vi "SECADO_JKI_v120.vi"() -> ()   [LabVIEW 2017] (continued)
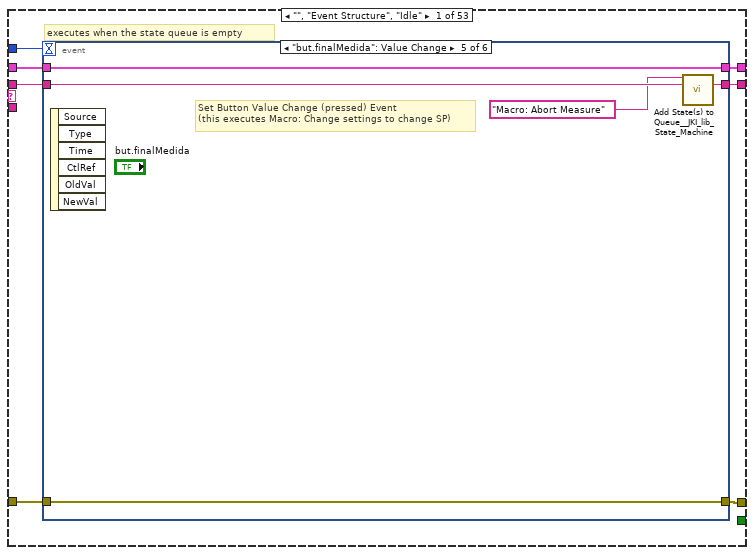
[diagram p2: hidden frame]
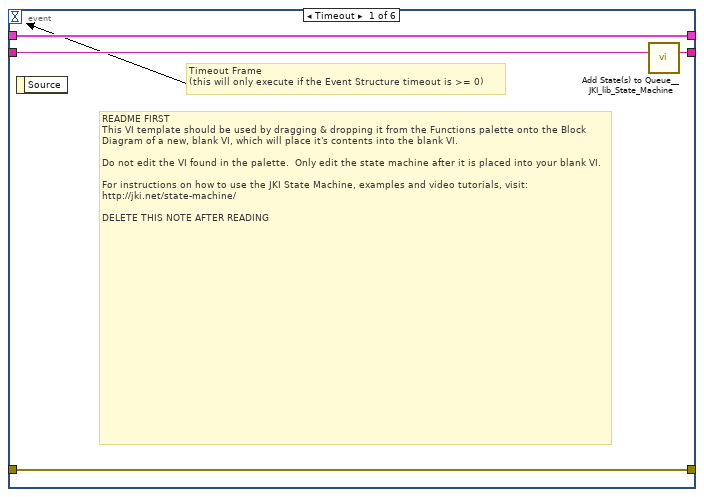
[diagram p3: hidden frame]
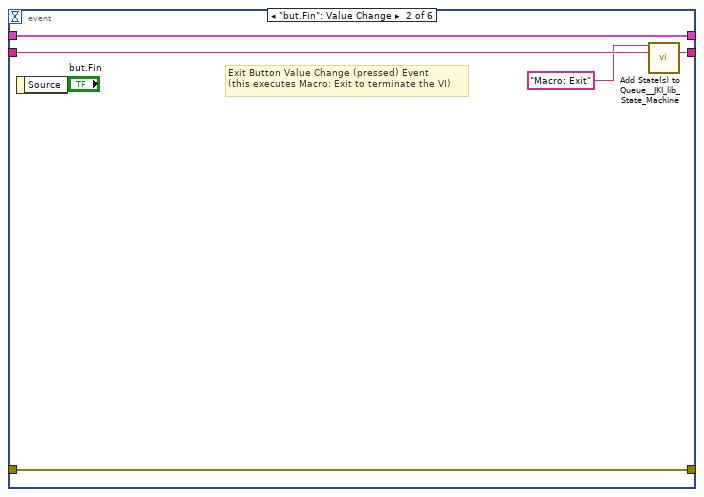
[diagram p4: hidden frame]
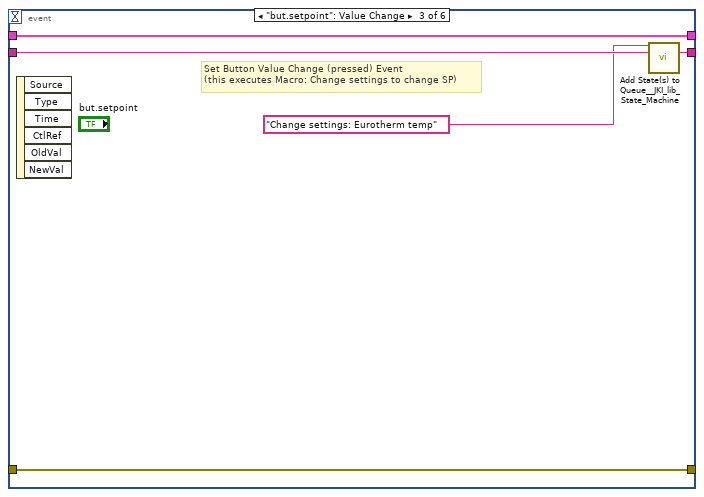
[diagram p5: hidden frame]
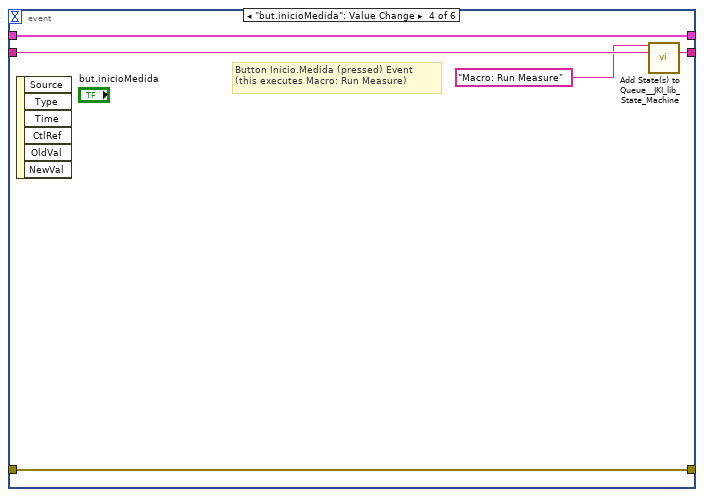
[diagram p6: hidden frame]
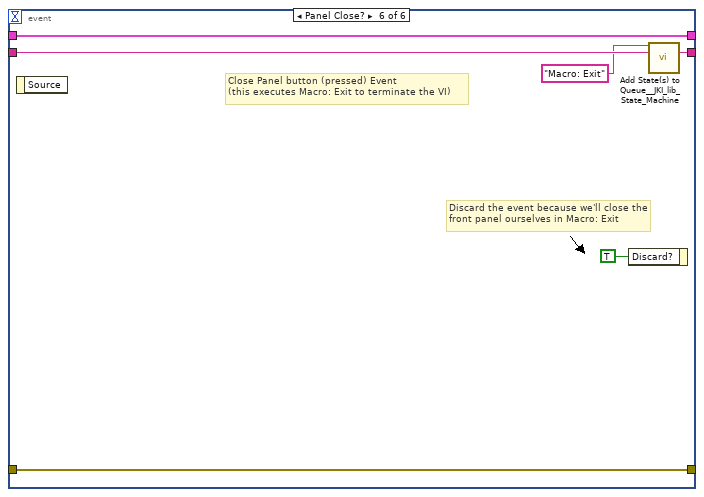
[diagram p7: hidden frame]
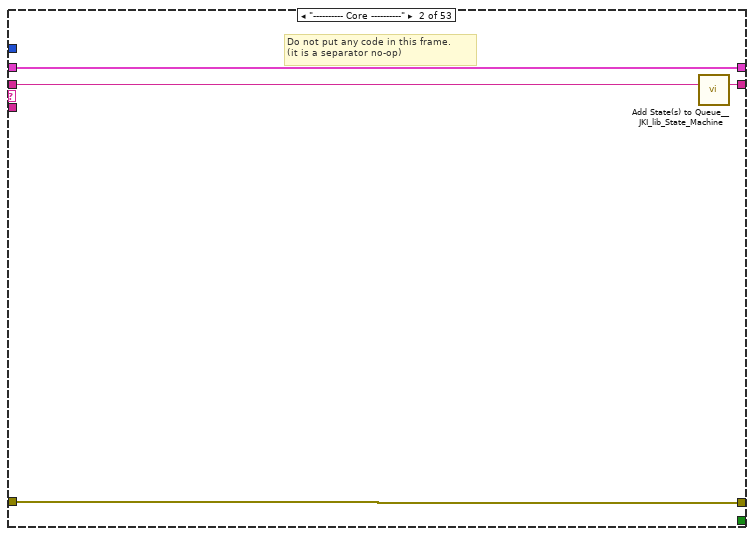
[diagram p8: hidden frame]
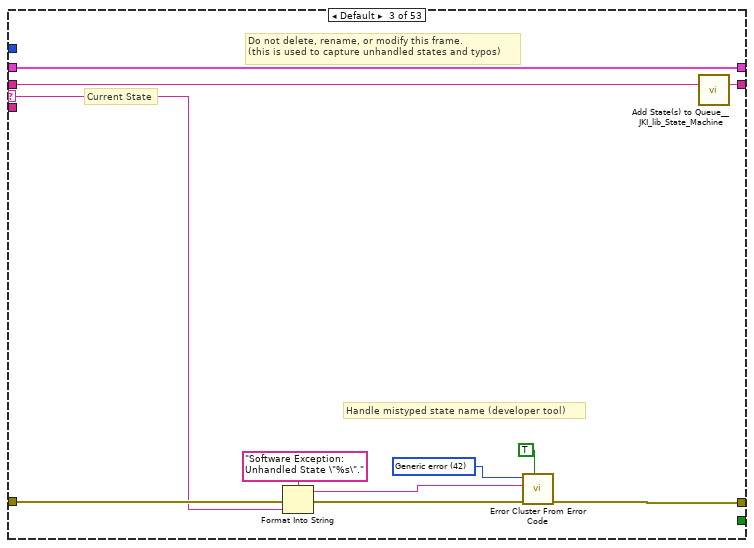
[diagram p9: hidden frame]
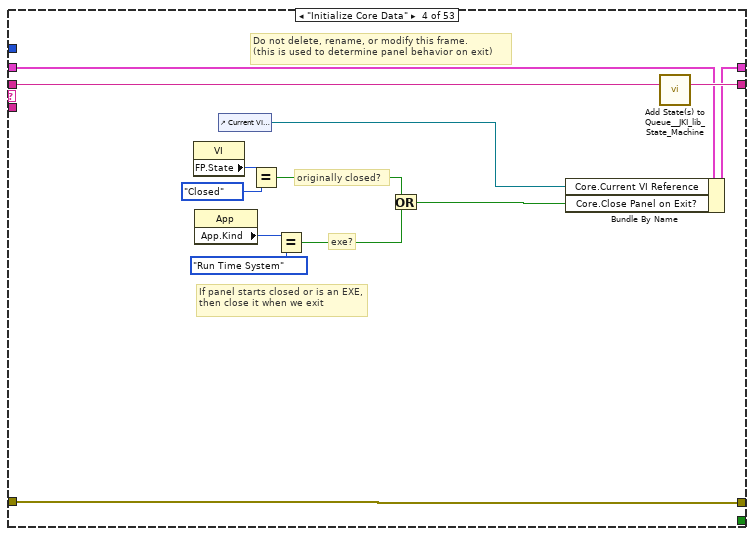
[diagram p10: hidden frame]
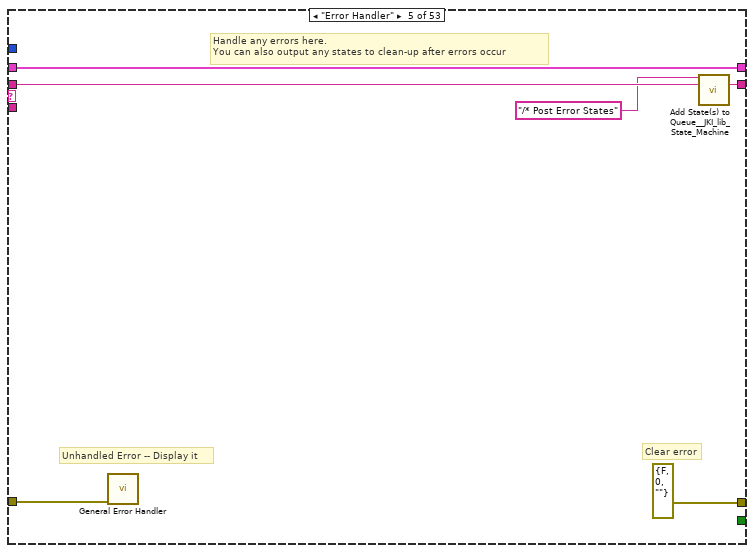
[diagram p11: hidden frame]
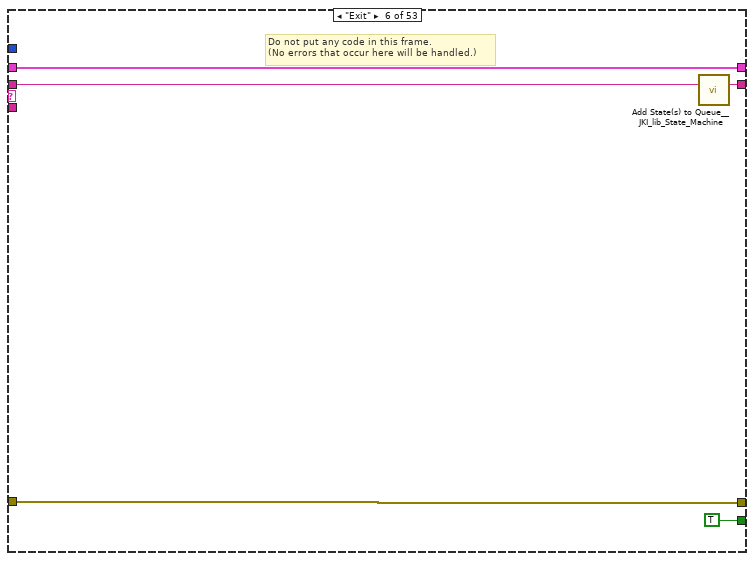
[diagram p12: hidden frame]
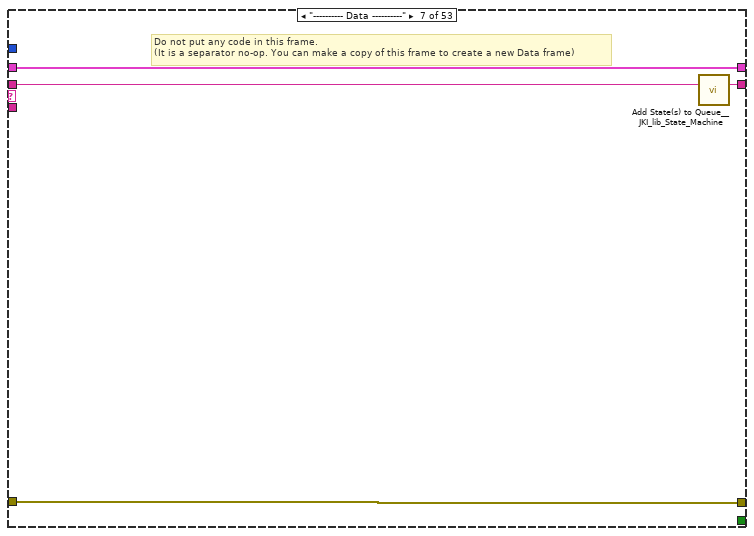
[diagram p13: hidden frame]
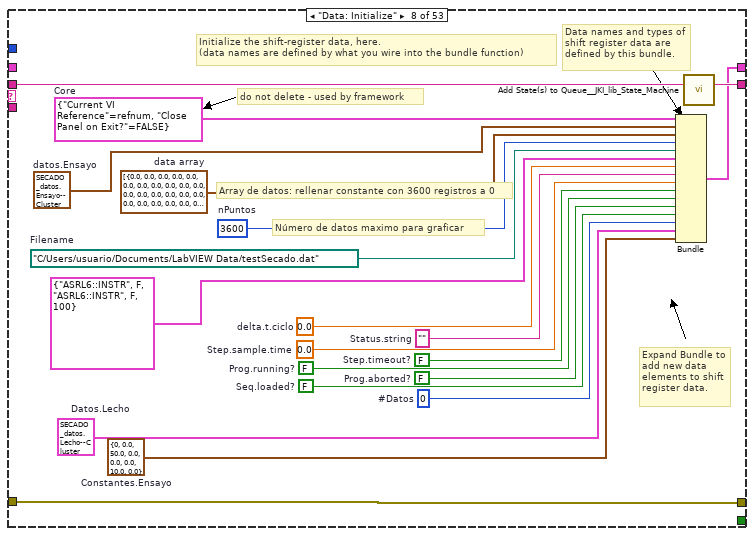
[diagram p14: hidden frame]
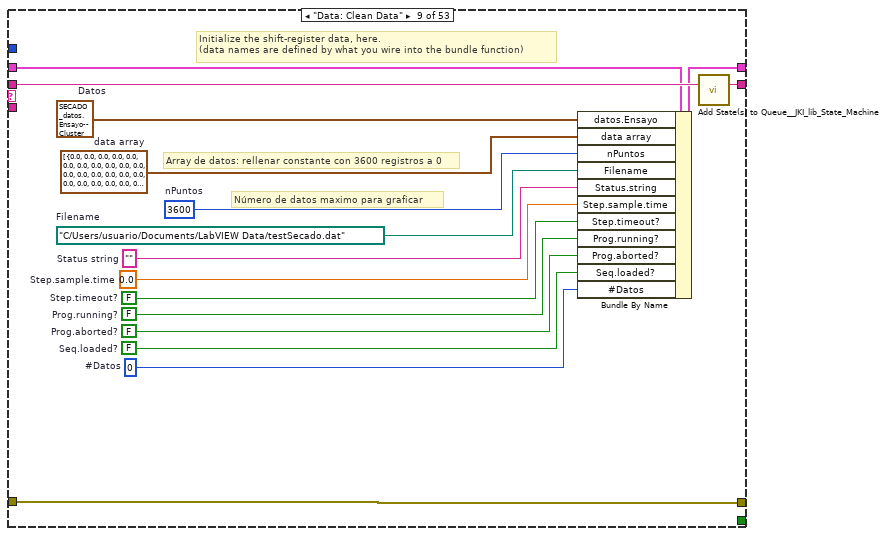
[diagram p15: hidden frame]
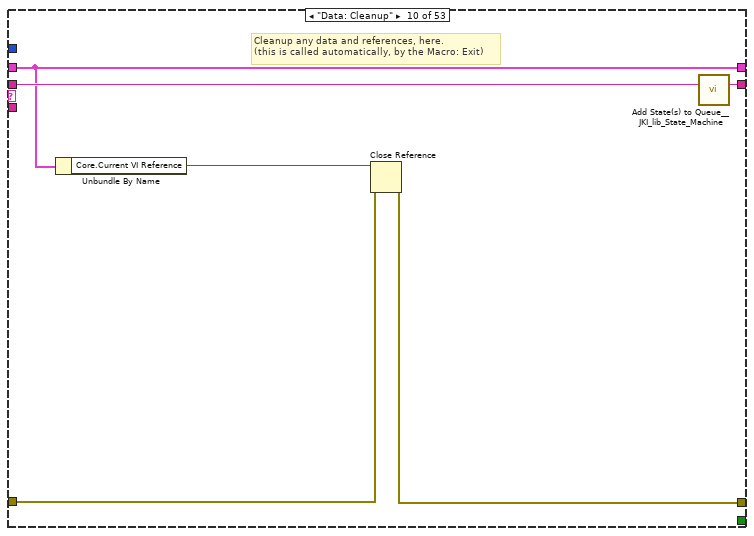
[diagram p16: hidden frame]
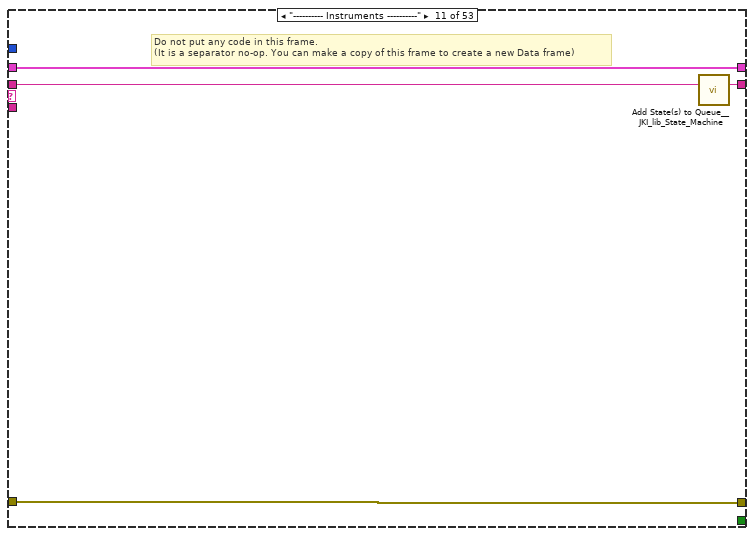
[diagram p17: hidden frame]
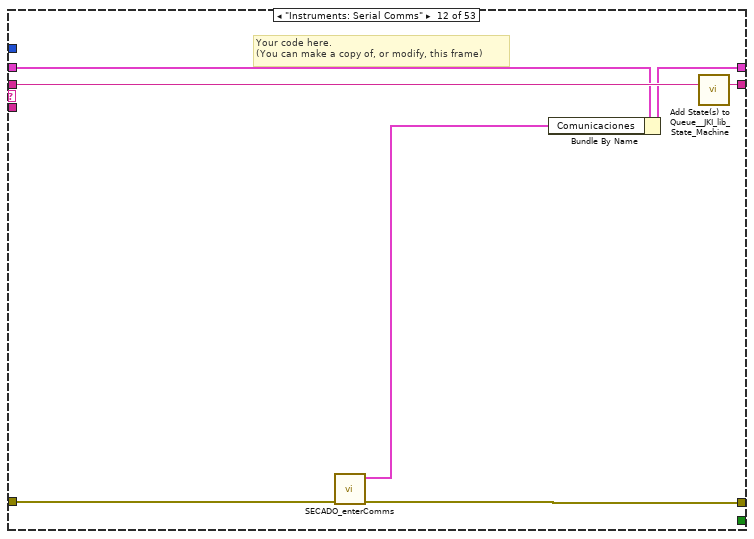
[diagram p18: hidden frame]
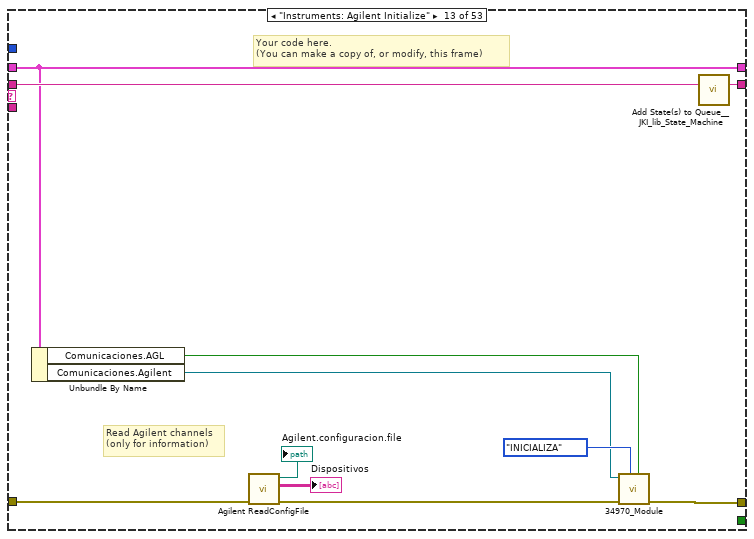
[diagram p19: hidden frame]
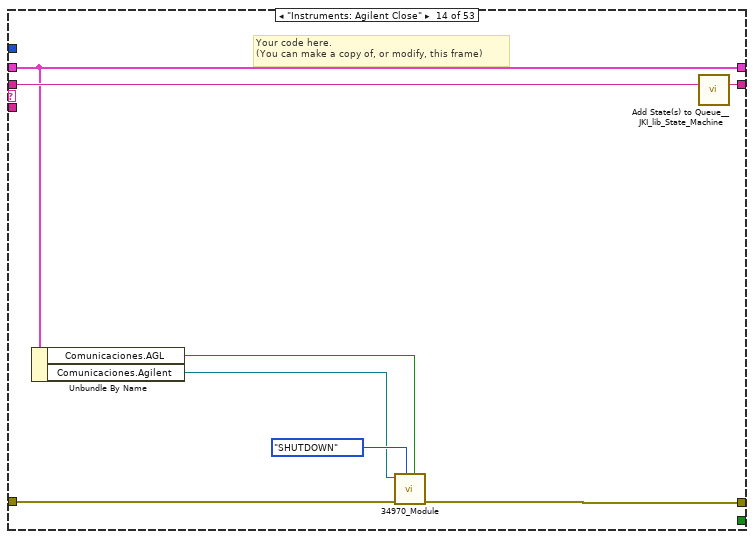
[diagram p20: hidden frame]
        n146 = Build Array(w405, w404, w403, w402) -> (→"EUROTHERM":cluster{dbl[], dbl[]}[])
        n147 = Build Array(w401, w400) -> (→"CAUDAL":cluster{dbl[], dbl[]}[])
        n148 = Build Array(w399) -> (→"POTENCIA CALEFACCION":cluster{dbl[], dbl[]}[])
        n149 = Build Array(w396, w395) -> (→"Q CEDIDO Y ABSORBIDO":cluster{dbl[], dbl[]}[])
        n150 = Build Array(w370, w369) -> (→"HUMEDAD":cluster{dbl[], dbl[]}[])
        n151 = Build Array(w368) -> (→"PRES_DIF":cluster{dbl[], dbl[]}[])
        n152 = Build Array(w388, w374, w373, w372, w371) -> (→"TEMPERATURA":cluster{dbl[], dbl[]}[])
        n153 = Build Array(w367, w360, w359) -> (→"VELOCIDAD AIRE":cluster{dbl[], dbl[]}[])
        n154 = Bundle By Name(cluster=w366, "data array"=w407) -> (w408:T19)
        n155 = call <vilib>:"Add State(s) to Queue__JKI_lib_State_Machine.vi"("State(s) in (\"\")"=w427) -> ("States Out"=w426:string)  [unwired: 14 in]
      }
      frame "---------- Macro ----------" {
        # "Do not put any code in this frame.\n(It is a separator no-op. You can make a copy of this frame to create a new Macro frame)"
        n156 = call <vilib>:"Add State(s) to Queue__JKI_lib_State_Machine.vi"("State(s) in (\"\")"=w455) -> ("States Out"=w454:string)  [unwired: 14 in]
      }
      frame "Macro: Inicializar" {
        w462 = "Data: Initialize\nData: Clean Data\nInitialize Core Data\nUI: Initialize\nUI: Front Panel State >> Open\nMacro: Interlock\nUI: Update Meas Data\nUI: Update Graphics\nInstruments: Serial Comms\nInstruments: Agilent Initialize\nInstruments: Eurotherm Initialize"  # Data: Initialize Data: Clean Data Initialize Core Data UI: Initialize UI: Front Panel State >> Open Macro: Interlock UI: Update Meas Data UI: Update Graphics Instruments: Serial Comms Instruments: Agilent Initialize Instruments: Eurotherm Initialize
        # "Initialization Macro\n(This is called once, when the VI starts)"
        n157 = Bundle By Name(cluster=w457, "Prog.running?"=TRUE ("Prog. Running?"), "Prog.aborted?"=FALSE ("Prog. Aborted?"), "Seq.loaded?"=FALSE ("Seq. Loaded?"), "Status.string"="Ready to start...") -> (w456:T19)
        n158 = call <vilib>:"Add State(s) to Queue__JKI_lib_State_Machine.vi"("State(s) in Front (\"\")"=w462, "State(s) in (\"\")"=w465) -> ("States Out"=w464:string)  [unwired: 13 in]
      }
      frame "Macro: Run Measure" {
        # "Run Measure Macro\n(This is called once, when the VI starts)"
        n159 = Bundle By Name(cluster=w472, "Prog.running?"=TRUE ("Prog. Running?"), "Prog.aborted?"=FALSE ("Prog. Aborted?"), "Seq.loaded?"=FALSE ("Seq. Loaded?"), "Status.string"="Adquisition in progress...") -> (w470:T19)
        n160 = call <vilib>:"Add State(s) to Queue__JKI_lib_State_Machine.vi"("State(s) in Front (\"\")"="UI: Initialize\nMacro: Interlock\nFile: Filename\nTiming: Initialize Total Time\nTiming: Initialize Sample Time\nMacro: Next Meas Cycle", "State(s) in (\"\")"=w475) -> ("States Out"=w474:string)  [unwired: 13 in]
      }
      frame "Macro: Abort Measure" {
        # "Abort Measure Macro\n(This is called when abort buton is pressed)"
        n161 = Bundle By Name(cluster=w480, "Prog.running?"=FALSE ("Prog. Running?"), "Prog.aborted?"=TRUE ("Prog. Aborted?"), "Seq.loaded?"=FALSE ("Seq. Loaded?"), "Status.string"="Adquisition aborted...") -> (w479:T19)
        n162 = One Button Dialog(message="Measure aborted") -> ()  [unwired: 1 in, 1 out]
        n163 = call <vilib>:"Add State(s) to Queue__JKI_lib_State_Machine.vi"("State(s) in (\"\")"="// Data: Set Seq. Aborted Flag >> True\n// Macro: Interlock\n// IO: Dwell  // finish current step (remove to abort immediately)\n// Data: Set Running Step >> -1\n// UI: Update Table Selection\n// Data: Set Seq. Aborted Flag >> False\nMacro: Interlock") -> ("States Out"=w485:string)  [unwired: 14 in]
      }
      frame "Macro: Next Meas Cycle" {
        # "Initialization Macro\n(This is called once, when the VI starts)"
        n164 = Unbundle By Name(w489) -> ("#Datos"=w487:i32)
        n165 = Increment(x=w487) -> (x+1=w486:i32)
        "#.datos" <- w486
        n166 = Bundle By Name(cluster=w489, "#Datos"=w486) -> (w488:T19)
        n167 = call <vilib>:"Add State(s) to Queue__JKI_lib_State_Machine.vi"("State(s) in Front (\"\")"="Timing: Measure Total Time\nMacro: Take Data\nMacro: Calculate\nMacro: Interlock\nFile: Save Data\nUI: Update Meas Data\nUI: Update Graphics\nSampling: Check For Next Sample", "State(s) in (\"\")"=w493) -> ("States Out"=w492:string)  [unwired: 13 in]
      }
      frame "Macro: Take Data" {
        # "Initialization Macro\n(This is called once, when the VI starts)"
        n168 = call <vilib>:"Add State(s) to Queue__JKI_lib_State_Machine.vi"("State(s) in Front (\"\")"="Measure data: Agilent Temp.PT100\nMeasure data: Agilent Temp.TERMOPAR\nMeasure data: Agilent Pressure\nMeasure data: Agilent Humidity\nMeasure data: Eurotherm Temperature", "State(s) in (\"\")"=w498) -> ("States Out"=w497:string)  [unwired: 13 in]
      }
      frame "Macro: Calculate" {
        # "Initialization Macro\n(This is called once, when the VI starts)"
        n169 = call <vilib>:"Add State(s) to Queue__JKI_lib_State_Machine.vi"("State(s) in Front (\"\")"="Calculations: Calculos 1", "State(s) in (\"\")"=w503) -> ("States Out"=w502:string)  [unwired: 13 in]
      }
      frame "Macro: Interlock" {
        # "Initialization Macro\n(This is called once, when the VI starts)"
        n170 = call <vilib>:"Add State(s) to Queue__JKI_lib_State_Machine.vi"("State(s) in Front (\"\")"="UI: Update Status\nUI: Update Interlock", "State(s) in (\"\")"=w508) -> ("States Out"=w507:string)  [unwired: 13 in]
      }
      frame "Macro: Exit" {
        # "Exit Macro\n(This is called once, when the VI exits)"
        n171 = Unbundle By Name(w516) -> ("Core.Close Panel on Exit?"=w515:bool)
        n172 = One Button Dialog(message="Program stop") -> ()  [unwired: 1 in, 1 out]
        n173 = Select(t="UI: Front Panel State >> Close", s=w515, f="") -> (s? t:f=w512:string)
        n174 = call <vilib>:"Add State(s) to Queue__JKI_lib_State_Machine.vi"("State(s) in (\"\")"=w512, "State(s) at Back (\"\")"="Data: Cleanup\nExit") -> ("States Out"=w510:string)  [unwired: 13 in]
        n175 = call <vilib>:"Add State(s) to Queue__JKI_lib_State_Machine.vi"("State(s) in Front (\"\")"=w510, "State(s) in (\"\")"=w519) -> ("States Out"=w518:string)  [unwired: 13 in]
      }
      frame "---------- File ----------" {
        # "Template Separator\n(You can make a copy of, or modify, this frame)"
        n176 = call <vilib>:"Add State(s) to Queue__JKI_lib_State_Machine.vi"("State(s) in (\"\")"=w523) -> ("States Out"=w522:string)  [unwired: 14 in]
      }
      frame "File: Filename" {
        # "Al arrancar la medida:\nHumedad.lecho = Humedad_inicial"
        # "Initialize and save head data"
        # "Your code here.\n(You can make a copy of, or modify, this frame)"
        n177 = call "SECADO_enterEnsayo.vi"("error in (no error)"=w530) -> ("error out"=w532:errorcluster, "Datos.Lecho"=w525:T5, "Constantes.Ensayo"=w526:T6)  [unwired: 7 in, 1 out]
        "Constantes.Ensayo" <- w526
        "Datos.Lecho" <- w525
        n178 = Unbundle By Name(w525) -> ("Hum_ini, f1"=w524:dbl)
        n179 = call "File_Module.vi"("Command"=File_Module_Control."Initialize", "error in (no error)"=w532, "Datos.Lecho"=w525, "Constantes.Ensayo"=w526) -> ("error out"=w529:errorcluster, "selected path"=w527:path)  [unwired: 6 in]
        "Fichero" <- w527
        n180 = Bundle By Name(cluster=w533, "Constantes.Ensayo"=w526, "Datos.Lecho"=w525, "Filename"=w527, "datos.Ensayo.Humedad.lecho, f1"=w524) -> (w528:T19)
        n181 = call <vilib>:"Add State(s) to Queue__JKI_lib_State_Machine.vi"("State(s) in (\"\")"=w535) -> ("States Out"=w534:string)  [unwired: 14 in]
      }
      frame "File: Save Data" {
        # "Your code here.\n(You can make a copy of, or modify, this frame)"
        n182 = Get Date/Time String() -> (date string=→"Fecha":string, time string=→"Hora":string)  [unwired: 3 in]
        n183 = Unbundle By Name(w538) -> ("datos.Ensayo"=w539:T4)
        n184 = call "File_Module.vi"("Command"=File_Module_Control."Save Data", "error in (no error)"=w541, "Datos.Ensayo"=w539) -> ("error out"=w540:errorcluster)  [unwired: 7 in, 1 out]
        n185 = call <vilib>:"Add State(s) to Queue__JKI_lib_State_Machine.vi"("State(s) in (\"\")"=w544) -> ("States Out"=w543:string)  [unwired: 14 in]
      }
      frame "---------- Sampling ----------" {
        # "Template Separator\n(You can make a copy of, or modify, this frame)"
        n186 = call <vilib>:"Add State(s) to Queue__JKI_lib_State_Machine.vi"("State(s) in (\"\")"=w548) -> ("States Out"=w547:string)  [unwired: 14 in]
      }
      frame "Sampling: Check For Next Sample" {
        # "Your code here.\n(You can make a copy of, or modify, this frame)"
        n187 = Unbundle By Name(w554) -> ("Step.timeout?"=w552:bool)
        n188 = Select(t="Timing: Initialize Sample Time\nMacro: Next Meas Cycle", s=w552, f="Idle  //Calls event structure\nTiming: Measure Sample Time\nSampling: Check For Next Sample // Come back here") -> (s? t:f=w550:string)
        n189 = call <vilib>:"Add State(s) to Queue__JKI_lib_State_Machine.vi"("State(s) in Front (\"\")"=w550, "State(s) in (\"\")"=w556) -> ("States Out"=w555:string)  [unwired: 13 in]
      }
      frame "---------- Measure data ----------" {
        # "Template Separator\n(You can make a copy of, or modify, this frame)"
        n190 = call <vilib>:"Add State(s) to Queue__JKI_lib_State_Machine.vi"("State(s) in (\"\")"=w560) -> ("States Out"=w559:string)  [unwired: 14 in]
      }
      frame "Measure data: Agilent Temp.PT100" {
        # "Agilent temperature readings code here.\n(You can make a copy of, or modify, this frame)"
        n191 = Unbundle By Name(w563) -> ("Comunicaciones.AGL"=w561:bool, "Comunicaciones.Agilent"=w562:refnum<visa-resource-name>)
        n192 = call "34970_Module.vi"("Agilent 34970A"=w561, "Command"=34970_Module_Control."LECTURA PT100", "error in (no error)"=w564, "VISA Agilent 34970A"=w562) -> ("error out"=w565:errorcluster, "TEMP.PT100"=w571:dbl[])  [unwired: 3 in, 3 out]
        n193 = Index Array(array=w571) -> (element #1=w569:dbl, element #2=w568:dbl, element #3=w567:dbl, element #4=w566:dbl)  [unwired: 4 in]
        n194 = Bundle By Name(cluster=w563, "datos.Ensayo.Temp.pt100.1, C"=w569, "datos.Ensayo.Temp.pt100.2, C"=w568, "datos.Ensayo.Temp.pt100.3, C"=w567, "datos.Ensayo.Temp.pt100.4, C"=w566) -> (w570:T19)
        n195 = call <vilib>:"Add State(s) to Queue__JKI_lib_State_Machine.vi"("State(s) in (\"\")"=w574) -> ("States Out"=w573:string)  [unwired: 14 in]
      }
      frame "Measure data: Agilent Temp.TERMOPAR" {
        # "Agilent temperature readings code here.\n(You can make a copy of, or modify, this frame)"
        n196 = Unbundle By Name(w581) -> ("Comunicaciones.AGL"=w579:bool, "Comunicaciones.Agilent"=w580:refnum<visa-resource-name>)
        n197 = call "34970_Module.vi"("Agilent 34970A"=w579, "Command"=34970_Module_Control."LECTURA TERMOPAR", "error in (no error)"=w582, "VISA Agilent 34970A"=w580) -> ("error out"=w583:errorcluster, "TEMP.TERMOPAR"=w575:dbl[])  [unwired: 3 in, 3 out]
        n198 = Index Array(array=w575) -> (element #1=w586:dbl, element #2=w585:dbl, element #3=w584:dbl, element #4=w578:dbl, element #5=w577:dbl, element #6=w576:dbl)  [unwired: 6 in]
        n199 = Bundle By Name(cluster=w581, "datos.Ensayo.Temp.termopar.5, C"=w586, "datos.Ensayo.Temp.termopar.6, C"=w585, "datos.Ensayo.Temperatura.ext, C"=w584, "datos.Ensayo.Temp.termopar.7, C"=w578, "datos.Ensayo.Temp.termopar.8, C"=w577, "datos.Ensayo.Temp.termopar.9, C"=w576) -> (w587:T19)
        n200 = call <vilib>:"Add State(s) to Queue__JKI_lib_State_Machine.vi"("State(s) in (\"\")"=w590) -> ("States Out"=w589:string)  [unwired: 14 in]
      }
      frame "Measure data: Agilent Pressure" {
        # "Agilent pressure readings code here.\n(You can make a copy of, or modify, this frame)"
        n201 = Unbundle By Name(w595) -> ("Comunicaciones.AGL"=w593:bool, "Comunicaciones.Agilent"=w594:refnum<visa-resource-name>)
        n202 = call "34970_Module.vi"("Agilent 34970A"=w593, "Command"=34970_Module_Control."LECTURA CAUDAL", "error in (no error)"=w596, "VISA Agilent 34970A"=w594) -> ("error out"=w597:errorcluster, "CAUDAL"=w591:dbl[])  [unwired: 3 in, 3 out]
        n203 = Index Array(array=w591) -> (element=w598:dbl)  [unwired: 1 in]
        n204 = Bundle By Name(cluster=w595, "datos.Ensayo.Q.caudal.vol, m3/h"=w598) -> (w599:T19)
        n205 = call <vilib>:"Add State(s) to Queue__JKI_lib_State_Machine.vi"("State(s) in (\"\")"=w601) -> ("States Out"=w600:string)  [unwired: 14 in]
      }
      frame "Measure data: Agilent Humidity" {
        # "Agilent humidity readings code here.\n(You can make a copy of, or modify, this frame)"
        n206 = Unbundle By Name(w606) -> ("Comunicaciones.AGL"=w604:bool, "Comunicaciones.Agilent"=w605:refnum<visa-resource-name>)
        n207 = call "34970_Module.vi"("Agilent 34970A"=w604, "Command"=34970_Module_Control."LECTURA HUMEDAD", "error in (no error)"=w607, "VISA Agilent 34970A"=w605) -> ("error out"=w608:errorcluster, "HUMEDAD"=w602:dbl[])  [unwired: 3 in, 3 out]
        n208 = Index Array(array=w602) -> (element #1=w610:dbl, element #2=w609:dbl)  [unwired: 2 in]
        n209 = Bundle By Name(cluster=w606, "datos.Ensayo.Humedad.rel.3, f1"=w610, "datos.Ensayo.Humedad.rel.4, f1"=w609) -> (w611:T19)
        n210 = call <vilib>:"Add State(s) to Queue__JKI_lib_State_Machine.vi"("State(s) in (\"\")"=w613) -> ("States Out"=w612:string)  [unwired: 14 in]
      }
      frame "Measure data: Eurotherm Temperature" {
        # "POTENCIA MAXIMA"
        # "Your code here.\n(You can make a copy of, or modify, this frame)"
        n211 = Unbundle By Name(w637) -> ("Comunicaciones.CDT"=w631:bool, "Comunicaciones.Eurotherm"=w632:refnum<visa-resource-name>, "Comunicaciones.#dec"=w617:T10)
        n212 = local read "Constantes.Ensayo"() -> (w616:T6)
        n213 = Unbundle By Name(w616) -> ("Voltaje_resist, vac"=w614:dbl, "Resistencia, ohm"=w615:dbl)
        n214 = call "Eurotherm_2023_Module.vi"("Eurotherm (T:Enable)"=w631, "Command"=Eurotherm_2023_Module."Initialize", "error in (no error)"=w636, "VISA resource name"=w632) -> ("error out"=w629:errorcluster)  [unwired: 5 in, 2 out]
        n215 = Square(x=w614) -> (x^2=w625:dbl)
        n216 = call "Eurotherm_2023_Module.vi"("Decimales"=w617, "Eurotherm (T:Enable)"=w631, "Command"=Eurotherm_2023_Module."Read data", "error in (no error)"=w629, "Address"=Address."Add 1", "VISA resource name"=w632) -> ("error out"=w628:errorcluster, "Eurotherm"=w627:T21)  [unwired: 3 in, 1 out]
        n217 = Divide(x=w625, y=w615) -> (x/y=w624:dbl)
        n218 = Unbundle By Name(w627) -> ("workingSP"=w621:dbl, "processVal"=w620:dbl, "workingOut"=w618:dbl)
        n219 = Multiply(x=w618, y=w624) -> (x*y=w623:dbl)
        n220 = Divide(x=w623, y=100.0) -> (x/y=w619:dbl)
        n221 = call "Eurotherm_2023_Module.vi"("Eurotherm (T:Enable)"=w631, "Command"=Eurotherm_2023_Module."Shutdown", "error in (no error)"=w628, "VISA resource name"=w632) -> ("error out"=w634:errorcluster)  [unwired: 5 in, 2 out]
        n222 = Bundle By Name(cluster=w637, "datos.Ensayo.P116.set.temp, C"=w621, "datos.Ensayo.P116.temperatura, C"=w620, "datos.Ensayo.P116.output, %"=w618, "datos.Ensayo.P116.output, W"=w619) -> (w633:T19)
        n223 = call <vilib>:"Add State(s) to Queue__JKI_lib_State_Machine.vi"("State(s) in (\"\")"=w640) -> ("States Out"=w639:string)  [unwired: 14 in]
      }
      frame "---------- Change settings ----------" {
        # "Template Separator\n(You can make a copy of, or modify, this frame)"
        n224 = call <vilib>:"Add State(s) to Queue__JKI_lib_State_Machine.vi"("State(s) in (\"\")"=w644) -> ("States Out"=w643:string)  [unwired: 14 in]
      }
      frame "Change settings: Eurotherm temp" {
        # "Your code here.\n(You can make a copy of, or modify, this frame)"
        n225 = Unbundle By Name(w654) -> ("datos.Ensayo.P116.set.temp, C"=w646:dbl, "Comunicaciones"=w651:T9, "Comunicaciones.CDT"=w653:bool, "Comunicaciones.Eurotherm"=w652:refnum<visa-resource-name>, "Comunicaciones.#dec"=w650:T10)
        n226 = Bundle By Name(cluster=T17 {"TargetSP"={"Ch1"=0.0}, "WorkingSP"={"Ch1"=0.0}, "Temperatura"={"Ch1"=0.0}, "RateSP"={"Ch1"=0.0}, "Potencia"={"Ch1"=0.0}, "Potencia max"={"Ch1"=0.0}} ("P116x1ch"), "RateSP.Ch1"=0.0, "TargetSP.Ch1"=w646) -> (w648:T17)
        n227 = call "Eurotherm_2023_Module.vi"("Eurotherm (T:Enable)"=w653, "Command"=Eurotherm_2023_Module."Initialize", "error in (no error)"=w655, "VISA resource name"=w652) -> ("error out"=w659:errorcluster)  [unwired: 5 in, 2 out]
        n228 = call "P116x1ch_WriteManual.vi"("P116x1ch"=w648, "Decimales"=w650, "error in (no error)"=w659, "Comunicaciones"=w651) -> ("error out"=w658:errorcluster)  [unwired: 5 in, 2 out]
        n229 = call "Eurotherm_2023_Module.vi"("Eurotherm (T:Enable)"=w653, "Command"=Eurotherm_2023_Module."Shutdown", "error in (no error)"=w658, "VISA resource name"=w652) -> ("error out"=w649:errorcluster)  [unwired: 5 in, 2 out]
        n230 = call <vilib>:"Add State(s) to Queue__JKI_lib_State_Machine.vi"("State(s) in (\"\")"=w661) -> ("States Out"=w660:string)  [unwired: 14 in]
      }
      frame "---------- Calculations ----------" {
        # "Template Separator\n(You can make a copy of, or modify, this frame)"
        n231 = call <vilib>:"Add State(s) to Queue__JKI_lib_State_Machine.vi"("State(s) in (\"\")"=w665) -> ("States Out"=w664:string)  [unwired: 14 in]
      }
      frame "Calculations: Calculos 1" {
        w669 = T2 {"Agua.evap, g/s"=0.0, "Hum.lecho, %"=1.0, "Q.aire.seco, W"=50.0, "Q.evaporacion, W"=230.0, "Porosidad"=60.0, "Vel.air.reactor, m/s"=1.0}  # Calculos.Ensayo
        # "Set Front Panel Open or Closed\n(Usage: \"UI: Front Panel State >> Open|Close\")"
        n232 = Unbundle By Name(w679) -> ("Datos.Lecho"=w676:T5, "Constantes.Ensayo"=w677:T6, "datos.Ensayo"=w678:T4)
        n233 = call "SECADO_calculos_2.vi"("error in (no error)"=w681, "datos.Ensayo.in"=w678, "Constantes.Ensayo"=w677, "Datos.Lecho"=w676) -> ("error out"=w680:errorcluster, "datos.Ensayo.out"=w668:T4)  [unwired: 6 in]
        n234 = Unbundle By Name(w668) -> ("Agua.evapor, g/s"=w670:dbl, "Humedad.lecho, f1"=w671:dbl, "Q.aire.seco, W"=w672:dbl, "Q.evaporacion, W"=w673:dbl, "Porosidad,"=w674:dbl, "Vel.air.reactor, m/s"=w675:dbl)
        n235 = Bundle By Name(cluster=w669, "Agua.evap, g/s"=w670, "Hum.lecho, %"=w671, "Q.aire.seco, W"=w672, "Q.evaporacion, W"=w673, "Porosidad"=w674, "Vel.air.reactor, m/s"=w675) -> (→"Calculos.Ensayo":T2)
        n236 = Bundle By Name(cluster=w679, "datos.Ensayo"=w668, "datos.Ensayo.Presion.abs.ext, Pa"="PRES_EXT, Pa") -> (w682:T19)
        n237 = call <vilib>:"Add State(s) to Queue__JKI_lib_State_Machine.vi"("State(s) in (\"\")"=w684) -> ("States Out"=w683:string)  [unwired: 14 in]
      }
    }
    n238 = call <userlib>:"Wait (ms)__ogtk.vi"("error in (no error)"=w8, "milliseconds to wait"="t.wait, ms") -> ("error out"=w6:errorcluster)  [unwired: 8 in, 1 out]
    n239 = Unbundle By Name(w6) -> ("status"=→"Error":bool)
  }
  "error out" <- w2
  n240 = flat-sequence {
    tunnel: w2 -> [_]
    frame #0 {
      n241 = Quit LabVIEW(quit? (T)=TRUE) -> ()
    }
  }
